vi "Initialize.vi"(8 "error in (no error)":errorcluster, 10 "Opciones puerto":T1={"baud rate (9600)"=9600, "data bits (8)"=8, "parity (0:none)"=enum."None"} {"data bits (8)" min=5 max=8 step=1}, 11 "Puerto Serial":refnum<visa-resource-name>) -> (0 "error out":errorcluster, 3 "VISA resource name out":refnum<visa-resource-name>)   [LabVIEW 2020, in "Control de MaP.lvlib"]
doc: "Establece la comunicación con el instrumento"
uses:
  Control de MaP.lvlib
  Controls/Com Port Options.ctl
  <vilib>/Instr/_visa.llb/VISA Flush IO Buffer Mask.ctl
  <vilib>/Instr/_visa.llb/VISA Set IO Buffer Mask.ctl
  <vilib>/Instr/_visa.llb/VISA Configure Serial Port (Instr).vi
panel:
  # "Centro de investigaciones en óptica.  ALL RIGHTS RESERVED."
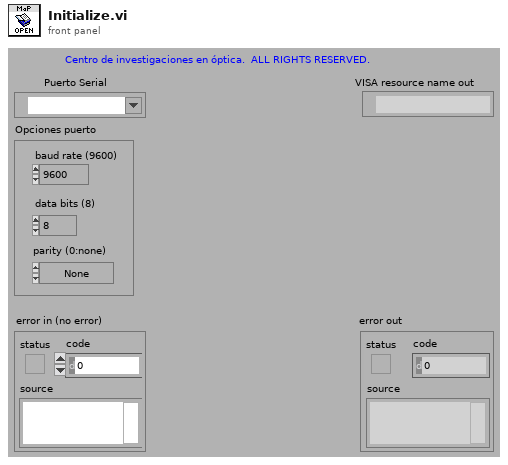
[diagram p1: front panel]
types:
  T1 = typedef "Control de MaP.lvlib/Com Port Options.ctl" = cluster{"baud rate (9600)":u32, "data bits (8)":u16, "parity (0:none)":enum16{"None", "Odd", "Even", "Mark", "Space"}}
  T2 = typedef "VISA Set IO Buffer Mask.ctl" = u16
  T3 = typedef "VISA Flush IO Buffer Mask.ctl" = u16
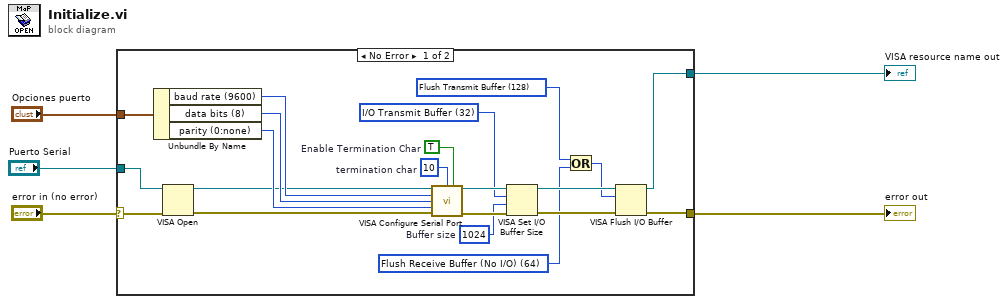
[diagram p0: block diagram]
diagram:
  n1 = case shown="No Error" "error in (no error)" {
    selector: "error in (no error)" -> [w10 w28]
    tunnel: "Puerto Serial" -> [w11 w27]
    tunnel: [w21 w27] -> w4
    tunnel: [w22 w28] -> w3
    tunnel: "Opciones puerto" -> [w26 _]
    frame No Error {
      w6 = TRUE  # Enable Termination Char
      w7 = u8 10  # termination char
      w12 = u32 1024  # Buffer size
      w13 = T2 32 items=["I/O Receive Buffer"=16, "I/O Transmit Buffer"=32, "I/O Receive and Transmit Buffer"=48] ("Mask")
      w14 = T3 64 items=["Flush Receive Buffer"=16, "Write Transmit Buffer to Device"=32, "Flush Receive Buffer (No I/O)"=64, "Flush Transmit Buffer"=128] ("Mask")
      w16 = T3 128 items=["Flush Receive Buffer"=16, "Write Transmit Buffer to Device"=32, "Flush Receive Buffer (No I/O)"=64, "Flush Transmit Buffer"=128] ("Mask")
      n2 = Unbundle By Name(w26) -> ("baud rate (9600)"=w25:u32, "data bits (8)"=w24:u16, "parity (0:none)"=w23:enum16{"None", "Odd", "Even", "Mark", "Space"})
      n3 = VISA Open(error in (no error)=w10, VISA resource name=w11) -> (VISA resource name=w8:refnum<visa-resource-name>, error out=w9:errorcluster)  [unwired: 3 in]
      n4 = call-poly "VISA Configure Serial Port"("VISA resource name"=w8, "termination char\n(0xA = '\\n' = LF)"=w7, "Enable Termination\nChar (T)"=w6, "baud rate (9600)"=w25, "data bits (8)"=w24, "parity (0:none)"=w23, "error in (no error)"=w9) -> ("VISA resource name out"=w20:refnum<visa-resource-name>, "error out"=w18:errorcluster)  [unwired: 7 in]
      n5 = VISA Set I/O Buffer Size(VISA resource name=w20, mask (16)=w13, size (4096)=w12, error in (no error)=w18) -> (VISA resource name out=w19:refnum<visa-resource-name>, error out=w17:errorcluster)
      n6 = Or(x=w16, y=w14) -> (x .or. y?=w15:T3)
      n7 = VISA Flush I/O Buffer(VISA resource name=w19, mask (16)=w15, error in (no error)=w17) -> (VISA resource name out=w21:refnum<visa-resource-name>, error out=w22:errorcluster)
    }
    frame Error {
    }
  }
  "VISA resource name out" <- w4
  "error out" <- w3
